vi "test Copy mixed integer cluster.vi"(8 "error in (no error)":errorcluster, 11 "TestCase in":refnum<class "Malleable Tests.lvclass">) -> (0 "error out":errorcluster, 3 "TestCase out":refnum<class "Malleable Tests.lvclass">)   [LabVIEW 2020, in "Memory Manager Tests.lvlib" / "Malleable Tests.lvclass"]
uses:
  Malleable Tests.lvclass
  Malleable Type Tests/Malleable Type Tests.lvclass
  C:/dev/illuminated-g/labview-memory-management-tools/Source/Classes/Pointer/Pointer.lvclass
  2ee8d6ef-e2c7-4ad2-b39a-c6cbc4b2dcd8.vi
  2ee8d6ef-e2c7-4ad2-b39a-c6cbc4b2dcd8.vi/48144062-09e8-44d7-a914-3b058f1e4a5b.vi
  Source/Classes/Pointer/Write U64.vi
  Source/Classes/Pointer/Write U32.vi
  Source/Classes/Pointer/Write U16.vi
  Source/Classes/Pointer/Check Null Pointer.vi
  Source/Classes/Pointer/Get Size.vi
  Source/Classes/Pointer/Get Address.vi
  <vilib>/addons/_JKI Toolkits/VI Tester/TestCase.llb/TestCase.lvclass
  Source/Classes/Pointer/Pointer.lvclass
  C:/dev/illuminated-g/labview-memory-management-tools/Tests/Memory Manager/Malleable Type Tests/Malleable Type Tests.lvclass
  C:/Program Files (x86)/National Instruments/LabVIEW 2020/vi.lib/addons/_JKI Toolkits/VI Tester/TestCase.llb/TestCase.lvclass
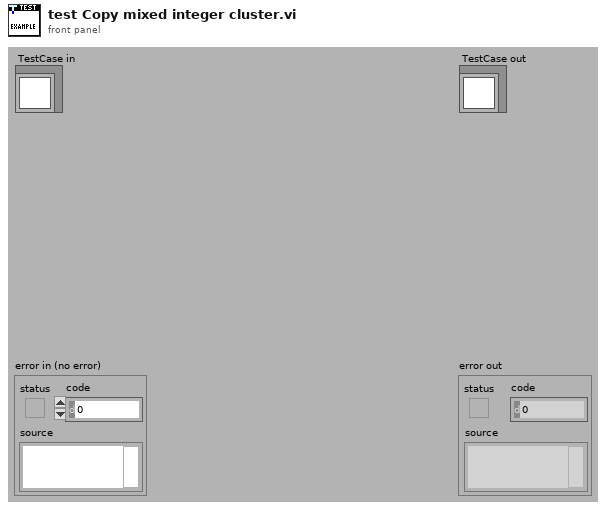
[diagram p1: front panel]
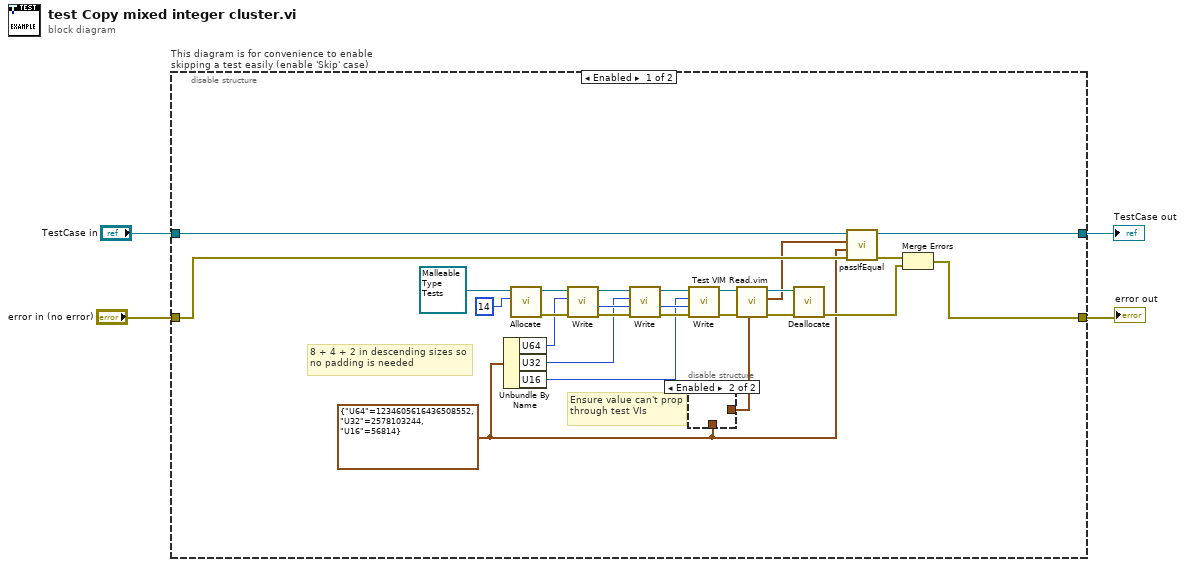
[diagram p0: block diagram]
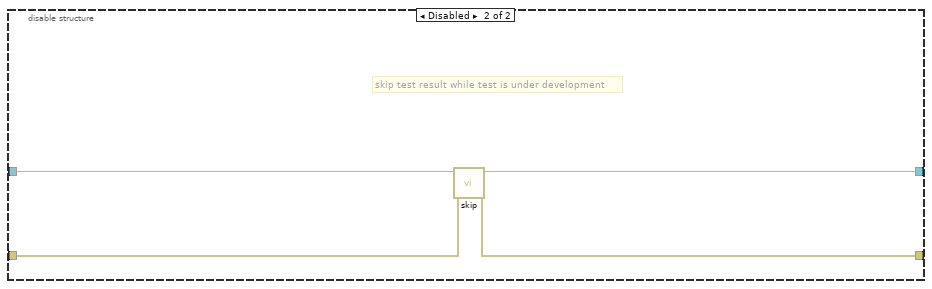
[diagram p3: hidden frame]
diagram:
  n1 = disable-structure "This diagram is for convenience to enable skipping a test easily (enable 'Skip' case)" shown="Enabled" {
    disable-tunnel: "TestCase in" -> [w10 w35]
    disable-tunnel: [w6 w33] -> w1
    disable-tunnel: [w12 w34] -> w3
    disable-tunnel: "error in (no error)" -> [w9 w32]
    frame Enabled {
      w7 = cluster{"U64":u64, "U32":u32, "U16":u16} {"U64"=1234605616436508552, "U32"=2578103244, "U16"=56814}
      # "Ensure value can't prop through test VIs"
      # "8 + 4 + 2 in descending sizes so no padding is needed"
      n2 = Unbundle By Name(w7) -> ("U64"=w26:u64, "U32"=w22:u32, "U16"=w18:u16)
      n3 = call "Allocate.vi"("size"=u64 14, "Pointer type"=refnum<class "Malleable Type Tests.lvclass"> refnum ("Memory Manager Tests.lvlib:Malleable Type Tests.lvclass")) -> ("error out"=w27:errorcluster, "Pointer out"=w28:refnum<class "Malleable Type Tests.lvclass">)  [unwired: 8 in]
      n4 = call-poly "Write.vi"("error in (no error)"=w27, "value"=w26, "Pointer in"=w28) -> ("error out"=w24:errorcluster, "offset + size"=w23:u64, "Pointer out"=w25:refnum<class "Malleable Type Tests.lvclass">)  [unwired: 5 in, 1 out]
      n5 = call-poly "Write.vi"("error in (no error)"=w24, "offset (0)"=w23, "value"=w22, "Pointer in"=w25) -> ("error out"=w20:errorcluster, "offset + size"=w19:u64, "Pointer out"=w21:refnum<class "Malleable Type Tests.lvclass">)  [unwired: 4 in, 1 out]
      n6 = call-poly "Write.vi"("error in (no error)"=w20, "offset (0)"=w19, "value"=w18, "Pointer in"=w21) -> ("error out"=w16:errorcluster, "Pointer out"=w17:refnum<class "Malleable Type Tests.lvclass">)  [unwired: 4 in, 2 out]
      n7 = disable-structure shown="Enabled" {
        disable-tunnel: w7 -> [w31 _]
        disable-tunnel: [w31 _] -> w15
        frame Disabled {
        }
        frame Enabled {
        }
      }
      n8 = call "Test VIM Read.vim"("Type"=w15, "error in (no error)"=w16, "Malleable Type Tests in"=w17) -> ("error out"=w14:errorcluster, "Value"=w8:cluster{"U64":u64, "U32":u32, "U16":u16}, "Malleable Type Tests out"=w13:refnum<class "Malleable Type Tests.lvclass">)  [unwired: 6 in]
      n9 = call "Deallocate.vi"("error in (no error)"=w14, "Pointer"=w13) -> ("error out"=w11:errorcluster)  [unwired: 8 in, 1 out]
      n10 = call-dynamic "passIfEqual.vi"("error in (no error)"=w9, "y"=w7, "x"=w8, "TestCase in"=w10) -> ("error out"=w5:errorcluster, "TestCase out"=w6:refnum<class "Malleable Tests.lvclass">)  [unwired: 6 in]
      n11 = Merge Errors(w5, w11) -> (w12:errorcluster)
    }
    frame Disabled {
      # "skip test result while test is under development"
      n12 = call <vilib>:"skip.vi"("error in (no error)"=w32, "TestCase in"=w35) -> ("error out"=w34:errorcluster, "TestCase out"=w33:refnum<class "Malleable Tests.lvclass">)  [unwired: 8 in]
    }
  }
  "error out" <- w3
  "TestCase out" <- w1
